vi "Get FW Path.vi"(0 "File":string(combo), 11 "Error In":errorcluster) -> (4 "Path":path, 15 "Error Out":errorcluster)   [LabVIEW 2021]
doc: "Returns the bootloader fw file path."
uses:
  <vilib>/Utility/config.llb/Read Key (String).vi
  <vilib>/Utility/config.llb/NI_LVConfig.lvlib
panel:
  # "Inputs"
  # "Outputs"
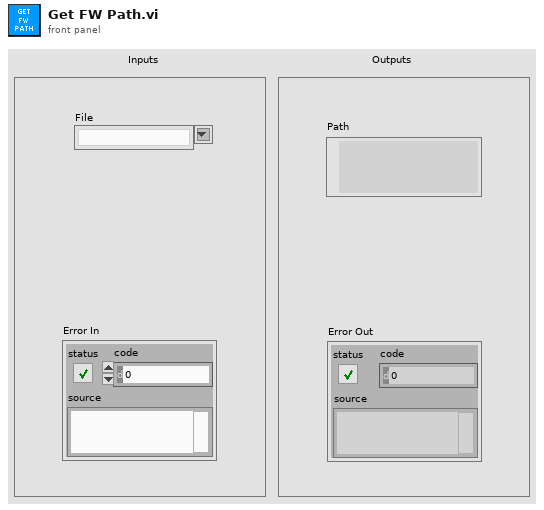
[diagram p1: front panel]
types:
  T1 = typedef "NI_LVConfig.lvlib/Config Data RefNum.ctl" = refnum<k1>
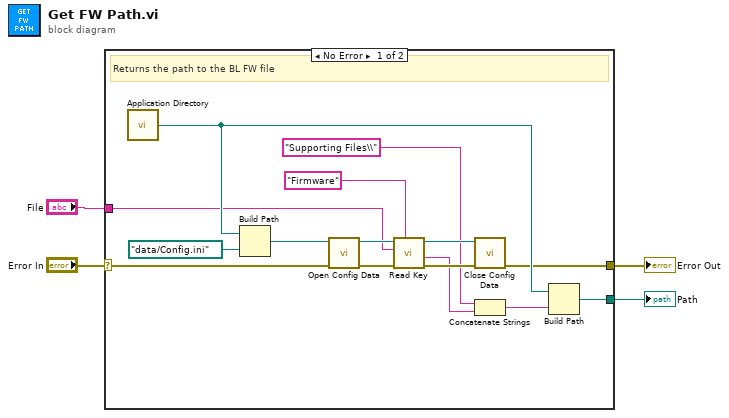
[diagram p0: block diagram]
diagram:
  n1 = case shown="No Error" "Error In" {
    selector: "Error In" -> [w11 w20]
    tunnel: [w10 w20] -> w3
    tunnel: [w9 _] -> w2
    tunnel: "File" -> [w5 _]
    frame No Error {
      # "Returns the path to the BL FW file"
      n2 = call <vilib>:"Application Directory.vi"() -> ("Application Directory"=w15:path)
      n3 = Build Path(base path=w15, name or relative path=path "data/Config.ini") -> (appended path=w13:path)
      n4 = call <vilib>:"Open Config Data.vi"("error in (no error)"=w11, "configuration file path"=w13) -> ("error out"=w18:errorcluster, "refnum"=w17:T1)  [unwired: 7 in, 1 out]
      n5 = call-poly <vilib>:"Read Key.vi"("section"="Firmware", "error in (no error)"=w18, "key"=w5, "refnum"=w17) -> ("error out"=w19:errorcluster, "value"=w7:string, "refnum out"=w16:T1)  [unwired: 4 in, 1 out]
      n6 = call <vilib>:"Close Config Data.vi"("error in (no error)"=w19, "refnum"=w16) -> ("error out"=w10:errorcluster)  [unwired: 8 in, 1 out]
      n7 = Concatenate Strings("Supporting Files\\" ("string"), w7) -> (w8:string)
      n8 = Build Path(base path=w15, name or relative path=w8) -> (appended path=w9:path)
    }
    frame Error {
      # "Can't start due to error"
    }
  }
  "Error Out" <- w3
  "Path" <- w2
